vi "Render.vi"(8 "error in (no error)":errorcluster, 10 "String in":string, 11 "DefinitionList in":refnum<class "DefinitionList.lvclass">) -> (0 "error out":errorcluster, 2 "String out":string, 3 "DefinitionList out":refnum<class "DefinitionList.lvclass">)   [LabVIEW 2021, in "LvMarkdown.lvlib" / "DefinitionList.lvclass"]
uses:
  DefinitionList.lvclass
  DefinitionList.lvclass/DefinitionList.ctl
  GetTerm.vi
  GetDefinition.vi
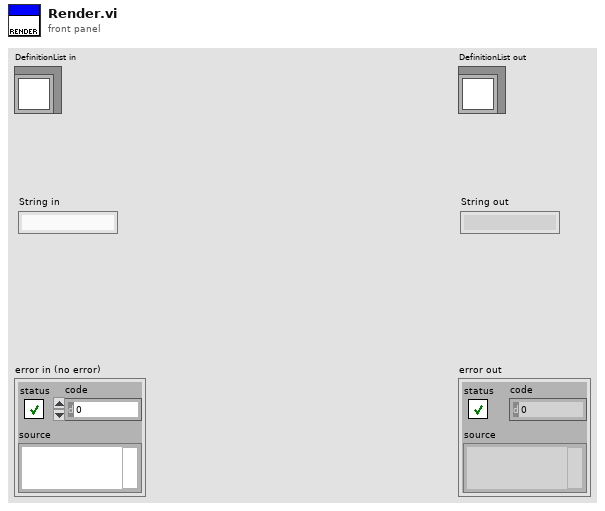
[diagram p1: front panel]
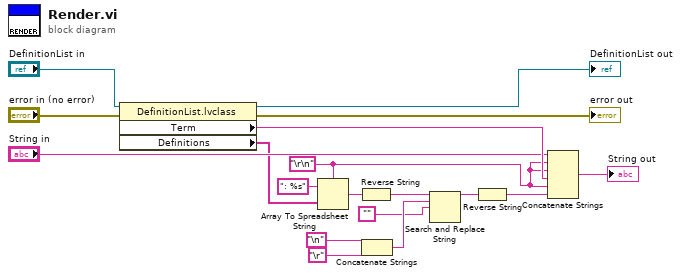
[diagram p0: block diagram]
diagram:
  w7 = "\r\n"
  n1 = property class="DefinitionList.lvclass"(reference="DefinitionList in", error in="error in (no error)") -> (reference out=→"DefinitionList out":refnum<class "DefinitionList.lvclass">, error out=→"error out":errorcluster, "Term"=w14:string, "Definitions"=w11:string[])
  n2 = Array To Spreadsheet String(delimiter (Tab)=w7, array=w11, 3:": %s" ("format string")) -> (spreadsheet string=w9:string)
  n3 = Reverse String(1:w9) -> (0:w8:string)
  n4 = Concatenate Strings("\n", "\r") -> (w3:string)
  n5 = Search and Replace String(input string=w8, search string=w3, replace string="") -> (result string=w6:string)  [unwired: 5 in, 3 out]
  n6 = Reverse String(1:w6) -> (0:w5:string)
  n7 = Concatenate Strings("String in", w7, w7, w14, w7, w5) -> (→"String out":string)
